vi "Server Exc_table.vi"(11 "BR":T1) -> (3 "appended array":string[](array[string]))   [LabVIEW 2014]
uses:
  Type'def/BR Exchange(Romte).ctl
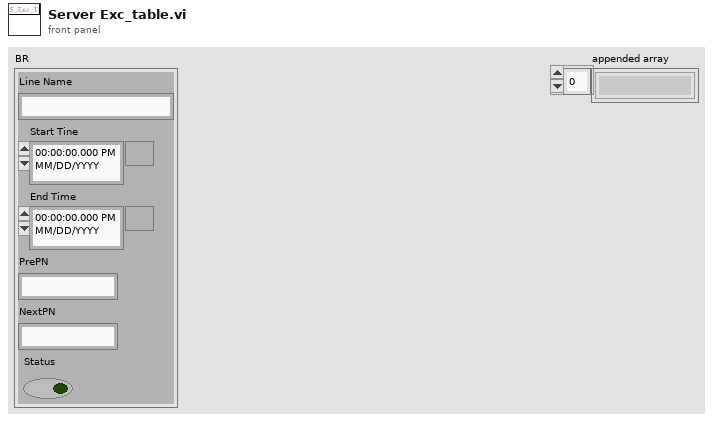
[diagram p1: front panel]
types:
  T1 = typedef "BR Exchange(Romte).ctl" = cluster{"Line Name":string, "Start Tine":timestamp, "End Time":timestamp, "PrePN":string, "NextPN":string, "Status":bool}
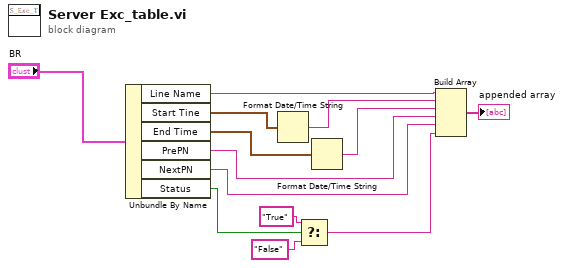
[diagram p0: block diagram]
diagram:
  n1 = Unbundle By Name("BR") -> ("Line Name"=w10:string, "Start Tine"=w12:timestamp, "End Time"=w11:timestamp, "PrePN"=w7:string, "NextPN"=w6:string, "Status"=w5:bool)
  n2 = Format Date/Time String(seconds (now)=w12) -> (date/time string=w9:string)  [unwired: 2 in]
  n3 = Select(t="True", s=w5, f="False") -> (s? t:f=w3:string)
  n4 = Format Date/Time String(seconds (now)=w11) -> (date/time string=w8:string)  [unwired: 2 in]
  n5 = Build Array(w10, w9, w8, w7, w6, w3) -> (→"appended array":string[])
